vi "CALC_FSIM_STAT.vi"(0 "VISA IN":refnum<visa-resource-name>, 1 "Fixturing ON/OFF":bool, 5 "error in":errorcluster, 7 "Channel":i32) -> (14 "VISA Out":refnum<visa-resource-name>, 19 "error out":errorcluster)   [LabVIEW 2018, in "PNA-X.lvlib"]
doc: "CALCulate<cnum>:FSIMulator:STATe <bool> \n(Read-Write) Turns all three fixturing functions (de-embedding, port matching, impedance \nconversion) ON or OFF for all ports on the specified channel. Does not affect port extensions. \nNote: This command affects ALL measurements on the specified channel. \nParameters \n<cnum> Channel number of the measurement. There must be a selected measurement \non that channel. If unspecified, <cnum> is set to 1. \n<bool> Choose from: \nON or 1 - Turns Fixturing ON \nOFF or 0 - Turns Fixturing OFF \nExamples CALC:FSIM:STAT 1 \ncalculate2:fsimulator:state 0 \nQuery Syntax CALCulate<cnum>:FSIMulator:STATe? \nReturn Type Boolean \nDefault OFF \n1514\n\n1515\n\nCalculate:Function Commands \nClick on a blue keyword to view the command details. \nSee Also \nExample Programs \nLearn about Trace Statistics \nSynchronizing the PNA and Controller \nSCPI Command Tree \nCritical Note: CALCulate commands act on the selected measurement. You can select one \nmeasurement for each channel using Calc:Par:Select"
uses:
  PNA-X.lvlib
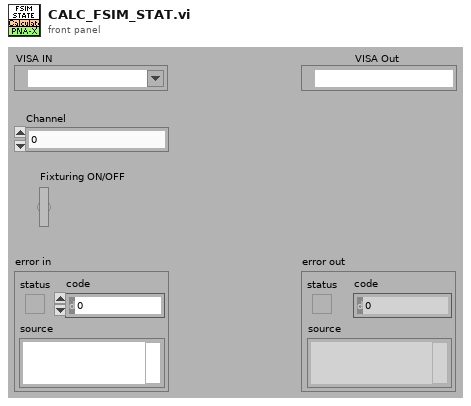
[diagram p1: front panel]
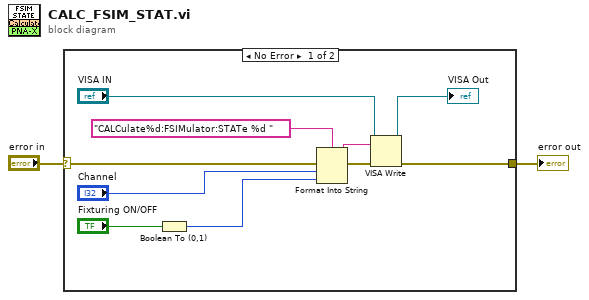
[diagram p0: block diagram]
diagram:
  n1 = case shown="No Error" "error in" {
    selector: "error in" -> [w12 w13]
    tunnel: [w7 w13] -> w1
    frame No Error {
      n2 = Boolean To (0,1)(Boolean="Fixturing ON/OFF") -> (0, 1=w3:i16)
      n3 = Format Into String(format string="CALCulate%d:FSIMulator:STATe %d " ("Cmdline"), error in=w12, "Channel", w3) -> (resulting string=w10:string, error out=w11:errorcluster)  [unwired: 1 in]
      n4 = VISA Write(VISA resource name="VISA IN", write buffer=w10, error in (no error)=w11) -> (VISA resource name out=→"VISA Out":refnum<visa-resource-name>, error out=w7:errorcluster)  [unwired: 1 out]
    }
    frame Error {
    }
  }
  "error out" <- w1
